vi "Search DAQ.vi"() -> (6 "Dev":tag, 7 "ProductType":string, 9 "isDevExist？":bool)   [LabVIEW 2016]
uses:
  <resource>/objmgr/daqmx.rc
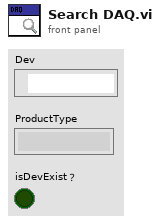
[diagram p1: front panel]
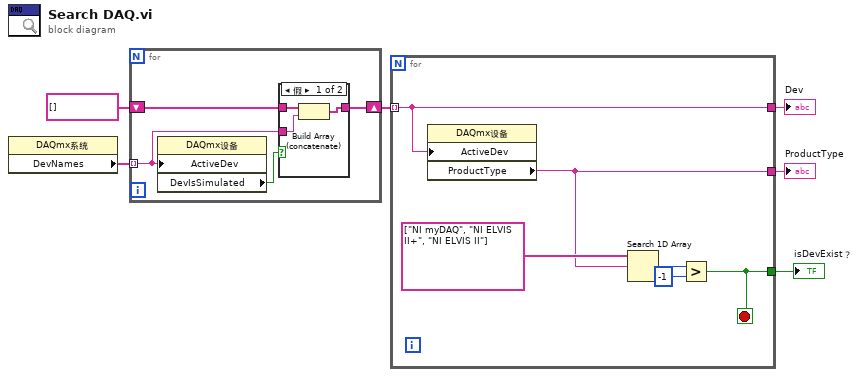
[diagram p0: block diagram]
diagram:
  n1 = property class="DAQmx系统"() -> ("DevNames"=w6:tag[])  [unwired: 2 in, 2 out]
  n2 = for {
    tunnel: w6 -> [w9] mode=indexing
    shift-right: [w7] -> w4
    shift-left: tag[] [] ("DevNames") -> [w8]
    n3 = property class="DAQmx设备"("ActiveDev"=w9) -> ("DevIsSimulated"=w10:bool)  [unwired: 2 in, 2 out]
    n4 = case shown="假" w10 {
      tunnel: w9 -> [w13 _]
      tunnel: w8 -> [w12 w14]
      tunnel: [w11 w14] -> w7
      frame False {
        n5 = Build Array (concatenate)(w12, w13) -> (w11:tag[])
      }
      frame True {
      }
    }
  }
  n6 = for {
    tunnel: [w15] -> w2
    tunnel: [w18] -> w3
    tunnel: w4 -> [w20] mode=indexing
    tunnel: [w20] -> w1
    stop <- w15 stop-if-true
    n7 = property class="DAQmx设备"("ActiveDev"=w20) -> ("ProductType"=w18:string)  [unwired: 2 in, 2 out]
    n8 = Search 1D Array(1D array=string[] ["NI myDAQ", "NI ELVIS II+", "NI ELVIS II"], element=w18) -> (index of element=w17:i32)  [unwired: 1 in]
    n9 = Greater?(x=w17, y=-1) -> (0:w15:bool)
  }
  "Dev" <- w1
  "isDevExist？" <- w2
  "ProductType" <- w3
